vi "sound_processing2.vi"() -> ()   [LabVIEW 2019]
panel:
  out "size(s)":i32
  out "Waveform Graph 2":waveform(dbl)(graph)
  out "data":waveform(dbl)[](array[waveform])
  out "Waveform Graph":waveform(dbl)[](graph)
  in  "Path":path
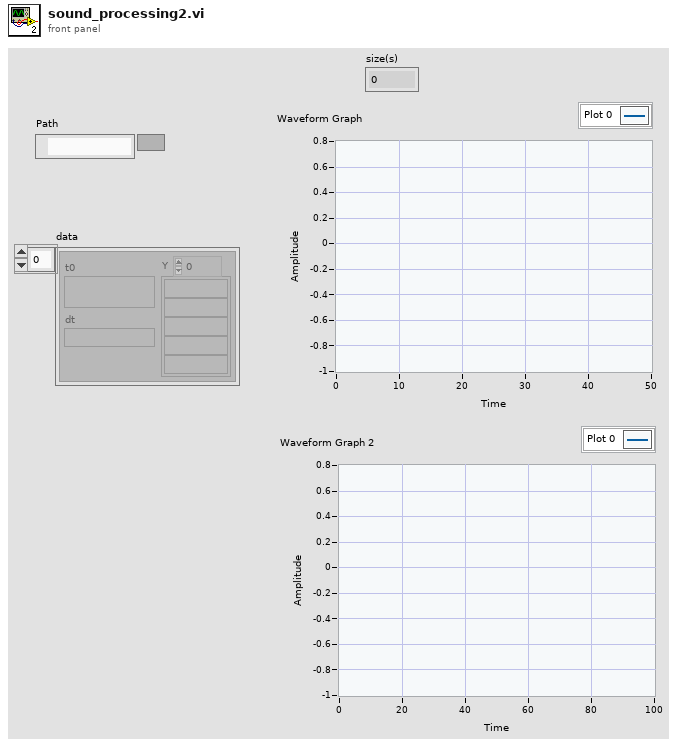
[diagram p1: front panel]
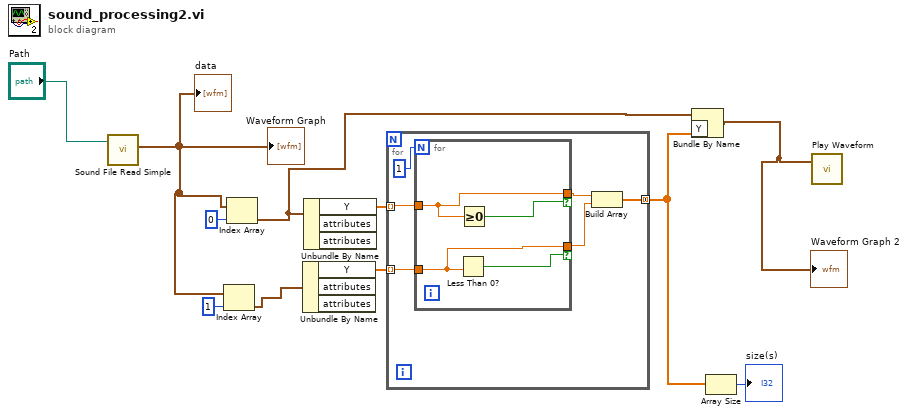
[diagram p0: block diagram]
diagram:
  n1 = call <vilib>:"Sound File Read Simple.vi"("path"="Path") -> ("data"=w7:waveform(dbl)[])  [unwired: 7 in, 3 out]
  "Waveform Graph" <- w7
  "data" <- w7
  n2 = Index Array(array=w7, index=1) -> (element=w5:waveform(dbl))
  n3 = Index Array(array=w7, index=0) -> (element=w8:waveform(dbl))
  n4 = Unbundle By Name(w5) -> ("Y"=w4:dbl[])  [unwired: 2 out]
  n5 = Unbundle By Name(w8) -> ("Y"=w9:dbl[])  [unwired: 2 out]
  n6 = for {
    tunnel: w9 -> [w17] mode=indexing
    tunnel: w4 -> [w16] mode=indexing
    tunnel: [w13] -> w2 mode=concatenating
    n7 = for {
      N: 1 -> [_]
      tunnel: w17 -> [w21]
      tunnel: [w21] -> w14 if=w20
      tunnel: w16 -> [w19]
      tunnel: [w19] -> w15 if=w18
      n8 = Less Than 0?(x=w19) -> (x < 0?=w18:bool)
      n9 = Greater Or Equal To 0?(x=w21) -> (x >= 0?=w20:bool)
    }
    n10 = Build Array(w14, w15) -> (w13:dbl[])
  }
  n11 = Bundle By Name(cluster=w8, "Y"=w2) -> (w3:waveform(dbl))
  "Waveform Graph 2" <- w3
  n12 = Array Size(array=w2) -> (size(s)=→"size(s)":i32)
  n13 = call "Play Waveform"("Data"=w3) -> ()  [unwired: 18 in, 1 out]
